vi "hcam_format_log_string.vi"(7 "sensor data in":T1) -> (8 "log string":string)   [LabVIEW 2020]
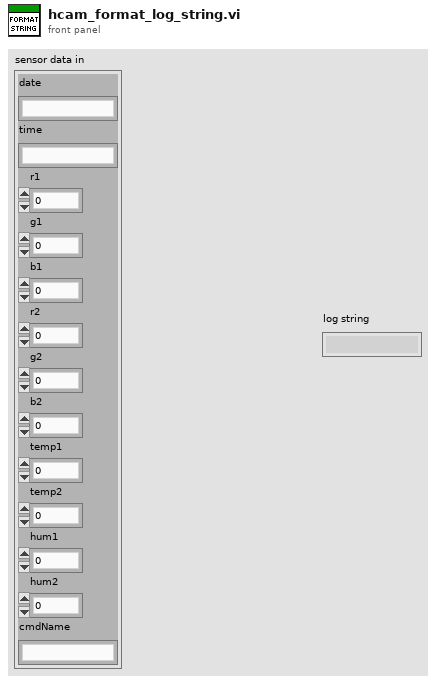
[diagram p1: front panel]
types:
  T1 = cluster{"date":string, "time":string, "r1":u8, "g1":u8, "b1":u8, "r2":u8, "g2":u8, "b2":u8, "temp1":sgl, "temp2":sgl, "hum1":sgl, "hum2":sgl, "cmdName":string}
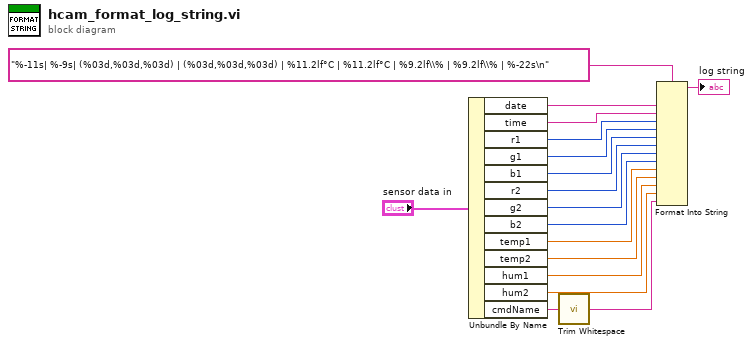
[diagram p0: block diagram]
diagram:
  n1 = Unbundle By Name("sensor data in") -> ("date"=w3:string, "time"=w4:string, "r1"=w16:u8, "g1"=w15:u8, "b1"=w14:u8, "r2"=w13:u8, "g2"=w12:u8, "b2"=w11:u8, "temp1"=w10:sgl, "temp2"=w9:sgl, "hum1"=w8:sgl, "hum2"=w7:sgl, "cmdName"=w2:string)
  n2 = call <vilib>:"Trim Whitespace.vi"("string"=w2) -> ("trimmed string"=w1:string)  [unwired: 1 in]
  n3 = Format Into String(format string="%-11s| %-9s| (%03d,%03d,%03d) | (%03d,%03d,%03d) | %11.2lf°C | %11.2lf°C | %9.2lf\\% | %9.2lf\\% | %-22s\n", w3, w4, w16, w15, w14, w13, w12, w11, w10, w9, w8, w7, w1) -> (resulting string=→"log string":string)  [unwired: 2 in, 1 out]
